vi "RT Main R1.vi"() -> ()   [LabVIEW 2018]
uses:
  Type Defs/Control Mode Type Def.ctl
  Type Defs/Sine Wave Inputs.ctl
  Type Defs/PID Inputs.ctl
  Type Defs/Measurement States.ctl
  <vilib>/Platform/TimedLoop/XDataNode/timing_clust.ctl
  <vilib>/Platform/TimedLoop/XDataNode/nitl_modes.ctl
  <vilib>/Platform/TimedLoop/XDataNode/wakeup.ctl
  <vilib>/FPGAPlugInAG/myRIO-1900/niLvFpga_Open_myRIO-1900.vi
  <vilib>/rvi/interface/common/dynamic/niFpgaDynamicAddResources.vi
  <vilib>/addons/control/pid/pid.llb/PID (DBL).vi
  <vilib>/Utility/error.llb/Error Cluster From Error Code.vi
  <vilib>/rvi/errors/niLvFpgaAdjustHostInterfaceError.vi
  <vilib>/FPGAPlugInAG/Dynamic/niLvFpga_Close_Dynamic.vi
  <vilib>/platform/TimedLoop/XDataNode/XDataNode.xnode
  <vilib>/rvi/interface/nirviOpenFPGA/nirviOpenFPGA.xnode
  FPGA Bitfiles/WattBalanceRev1_FPGATarget_FPGAMain_doRdIs9Lwbc.lvbitx
  FPGA/FPGA Main.vi
  <vilib>/rvi/interface/nirviReadWriteControl/nirviReadWriteControl.xnode
  <vilib>/rvi/interface/nirviCloseFPGA/nirviCloseFPGA.xnode
  <vilib>/rvi/interface/Simulation/niFpgaSimulationCallBeginRW.vi
  NiFpgaLv.dll
  <vilib>/Platform/TimedLoop/XDataNode/XDNodeRunTimeDep.lvlib
  <vilib>/addons/control/pid/NI_PID_pid.lvlib
panel:
  in  "Measure":bool
  out "Finished Late":bool
  in  "Amplifier On/Off":bool
  out "Voice Coil Input Voltage":dbl[](array[numeric]) format="%#.2g"
  out "Displacement (µm)":dbl[](array[numeric]) format="%#.2g"
  out "Voice Coil Back EMF":dbl[](array[numeric]) format="%#.2g"
  in  "PID Inputs":T1
  in  "Sine Wave\nInputs":T2
  in  "Manual Voice \nCoil Voltage":dbl format="%.2f"
  in  "Abort":bool
  in  "Control Mode":T3=enum."Manual"
  out "Chart":dynamicdata(graph) caption="Waveform Chart - dark"
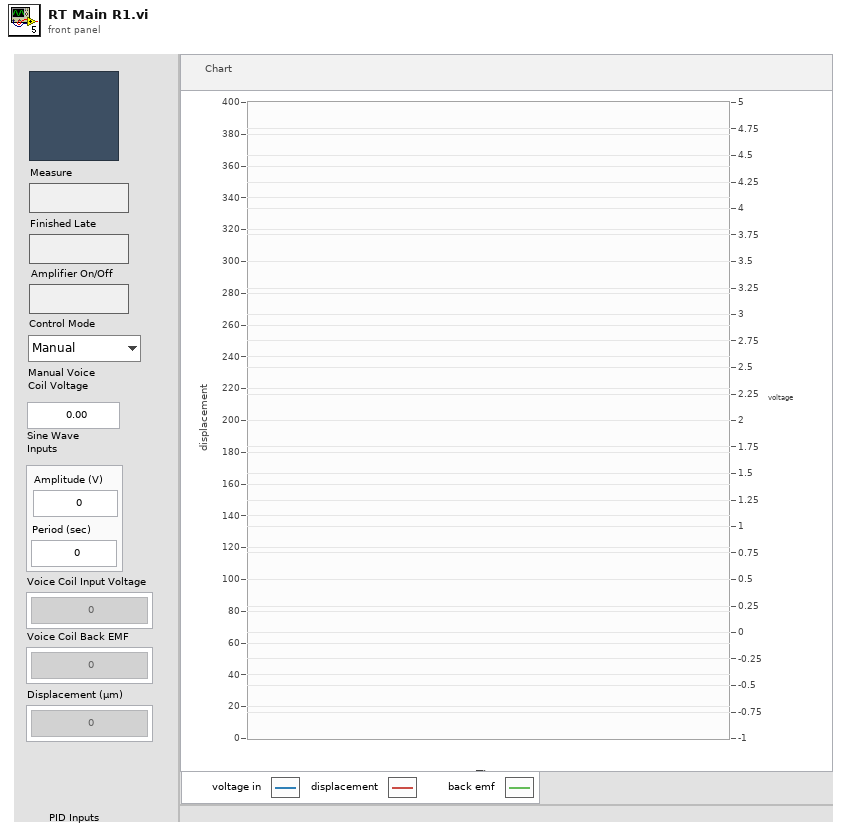
[diagram p1: front panel]
types:
  T1 = typedef "PID Inputs.ctl" = cluster{"PID":cluster{"Kp":dbl, "Ki":dbl, "Kd":dbl}, "Voltage Limits":cluster{"Max Voltage":dbl, "Min Voltage":dbl}, "Set Point (µm)":dbl}
  T2 = typedef "Sine Wave Inputs.ctl" = cluster{"Amplitude (V)":dbl, "Period (sec)":dbl}
  T3 = typedef "Control Mode Type Def.ctl" = enum16{"Sine", "PID", "Manual"}
  T4 = typedef "Measurement States.ctl" = enum16{"Idle", "Create File", "Collect Data", "Calculate", "Close"}
  T5 = typedef "XDNodeRunTimeDep.lvlib/timing_clust.ctl" = cluster{"Expected End [f-1]":u64, "Actual End [f-1]":u64, "Finished Late? [f-1]":bool, "Expected End [i-1]":u64, "Actual End [i-1]":u64, "Finished Late? [i-1]":bool, "Expected Start [i]":u64, "Actual Start [i]":u64, "Expected Start [f]":u64, "Actual Start [f]":u64, "Source Name":string, "Structure Name":string, "Period":i64, "Deadline":i64, "Offset":i64, "Start":i64, "Priority":i32, "Timeout":i32, "Mode":T6, "Wakeup Reason":T7, "Error":errorcluster, "Source Type":string, "Secondary Source Type":string, "Global End Time":u64, "Global Start Time":u64, "Frame Duration":u64, "Iteration Duration":u64, "Assigned CPU":i32, "I/O Scan Engine Mode":u32}
  T6 = typedef "XDNodeRunTimeDep.lvlib/nitl_modes.ctl" = enum32{"No Change", "Process missed periods, maintain original phase", "Discard missed periods, maintain original phase", "Process missed periods, ignore original phase", "Discard missed periods, ignore original phase"}
  T7 = typedef "XDNodeRunTimeDep.lvlib/wakeup.ctl" = enum32{"Normal", "Aborted", "Asynchronous wakeup", "Timing source error", "Timed loop error", "Timeout"}
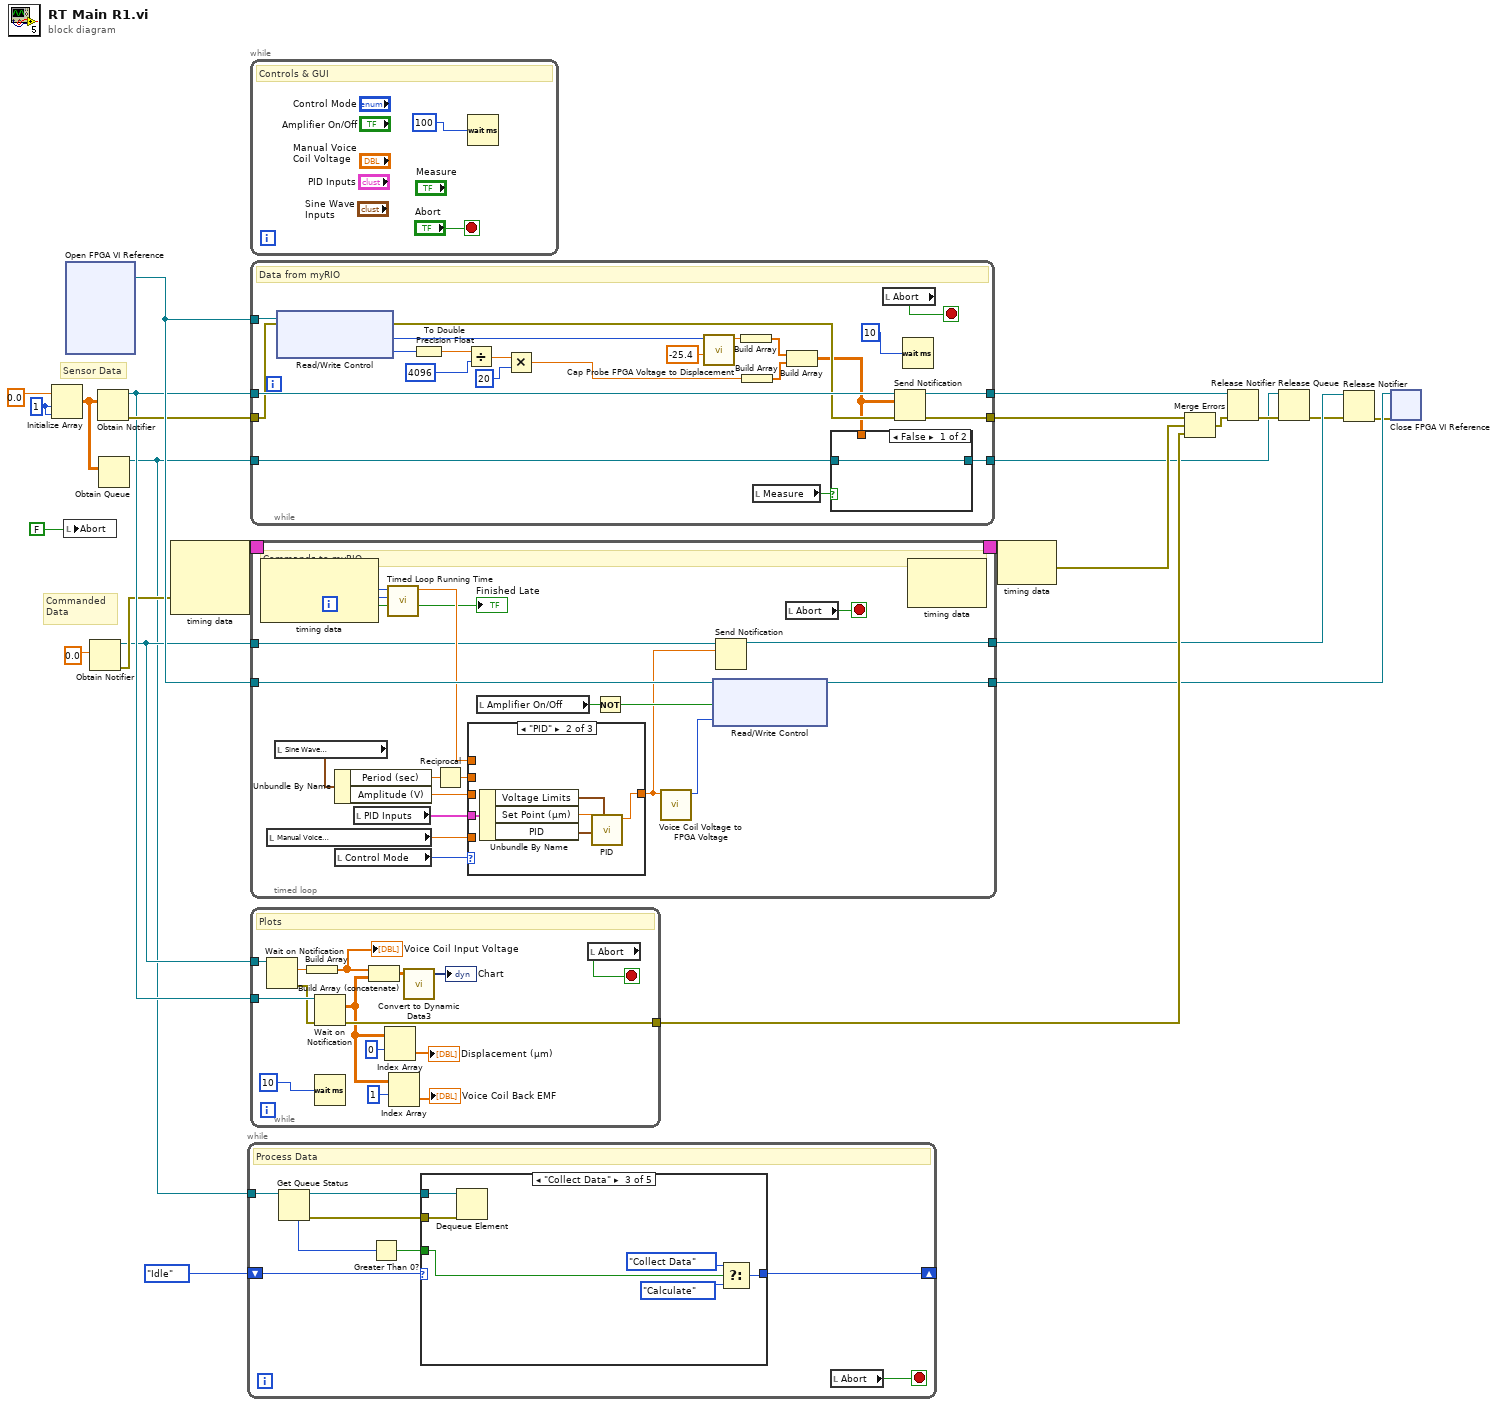
[diagram p0: block diagram]
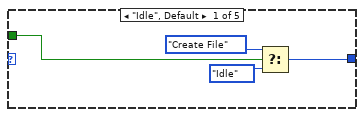
[diagram p2: hidden frame]
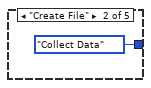
[diagram p3: hidden frame]
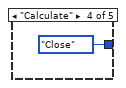
[diagram p4: hidden frame]
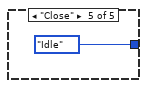
[diagram p5: hidden frame]
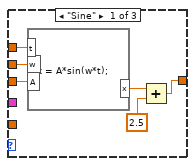
[diagram p6: hidden frame]
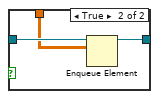
[diagram p8: hidden frame]
diagram:
  w21 = 1 ("dimension size")
  # "Commanded\nData"
  # "Sensor Data"
  n1 = Initialize Array(0.0, w21, w21) -> (w6:dbl[][])
  n2 = local write "Abort"(FALSE) -> ()
  n3 = xnode "Open FPGA VI Reference"() -> ("FPGA VI Reference Out"=w23:refnum<k20>)  [unwired: 2 in, 1 out]
  n4 = Obtain Notifier(notification data type=0.0) -> (notifier out=w11:refnum<notifier>, error out=w12:errorcluster)  [unwired: 3 in, 1 out]
  n5 = Obtain Notifier(notification data type=w6) -> (notifier out=w19:refnum<notifier>, error out=w20:errorcluster)  [unwired: 3 in, 1 out]
  n6 = Obtain Queue(element data type=w6) -> (queue out=w5:refnum<queue>)  [unwired: 4 in, 2 out]
  n7 = node-c288(w12) -> (w25:T5)  [unwired: 2 in]
  n8 = while {
    shift-right: [w28] -> _
    shift-left: Measurement_States."Idle" -> [w32]
    tunnel: w5 -> [w30]
    stop <- w33 stop-if-true
    # "Process Data"
    n9 = Get Queue Status(queue=w30) -> (queue out=w27:refnum<queue>, error out=w26:errorcluster, # elements in queue=w31:i32)  [unwired: 2 in, 5 out]
    n10 = Greater Than 0?(x=w31) -> (x > 0?=w29:bool)
    n11 = case shown="\"Collect Data\"" w32 {
      tunnel: w29 -> [w37 _ w44 _ _]
      tunnel: [w34 Measurement_States."Collect Data" w41 Measurement_States."Close" Measurement_States."Idle"] -> w28
      tunnel: w27 -> [_ _ w40 _ _]
      tunnel: w26 -> [_ _ w39 _ _]
      frame "Idle", Default {
        n12 = Select(t=Measurement_States."Create File", s=w37, f=Measurement_States."Idle") -> (s? t:f=w34:T4)
      }
      frame "Create File" {
      }
      frame "Collect Data" {
        n13 = Dequeue Element(queue=w40, error in (no error)=w39) -> ()  [unwired: 1 in, 4 out]
        n14 = Select(t=Measurement_States."Collect Data", s=w44, f=Measurement_States."Calculate") -> (s? t:f=w41:T4)
      }
      frame "Calculate" {
      }
      frame "Close" {
      }
    }
    n15 = local read "Abort"() -> (w33:bool)
  }
  n16 = while {
    stop <- "Abort" stop-if-true
    # "Controls & GUI"
    n17 = Wait (ms)(milliseconds to wait=100) -> ()  [unwired: 1 out]
  }
  n18 = while {
    tunnel: w23 -> [w70]
    tunnel: w19 -> [w63]
    tunnel: w20 -> [w62]
    tunnel: [w60] -> w14
    tunnel: [w59] -> w18
    tunnel: w5 -> [w51]
    tunnel: [w49] -> w2
    stop <- w67 stop-if-true
    # "Data from myRIO"
    n19 = xnode "Read/Write Control"("FPGA VI Reference In"=w70, "error in"=w62) -> ("error out"=w61:errorcluster, "Cap Probe Voltage"=w69:u16, "Read Coil"=w68:i16)  [unwired: 1 out]
    n20 = To Double Precision Float(number=w68) -> (double precision float=w57:dbl)
    n21 = Divide(x=w57, y=4096) -> (x/y=w55:dbl)
    n22 = Multiply(x=w55, y=20) -> (x*y=w53:dbl)
    n23 = call "Cap Probe FPGA Voltage to Displacement.vi"("Micrometers per Volt"=-25.4, "Cap Probe FPGA Voltage"=w69) -> ("Cap Probe Displacement"=w66:dbl)  [unwired: 9 in]
    n24 = Build Array(w66) -> (w65:dbl[])
    n25 = Build Array(w53) -> (w64:dbl[])
    n26 = local read "Measure"() -> (w52:bool)
    n27 = Build Array(w65, w64) -> (w50:dbl[][])
    n28 = case shown="False" w52 {
      tunnel: w51 -> [w72 w75]
      tunnel: w50 -> [_ w74]
      tunnel: [w72 w73] -> w49
      frame False {
      }
      frame True {
        n29 = Enqueue Element(queue=w75, element=w74) -> (queue out=w73:refnum<queue>)  [unwired: 2 in, 2 out]
      }
    }
    n30 = local read "Abort"() -> (w67:bool)
    n31 = Send Notification(notification=w50, notifier=w63, error in (no error)=w61) -> (notifier out=w60:refnum<notifier>, error out=w59:errorcluster)
    n32 = Wait (ms)(milliseconds to wait=10) -> ()  [unwired: 1 out]
  }
  n33 = timed-loop {
    timing: w25 -> [_]
    timing-out: [_] -> w24
    tunnel: w23 -> [w91]
    tunnel: [w86] -> w13
    tunnel: w11 -> [w79]
    tunnel: [w77] -> w9
    i -> [w83]
    stop <- w90 stop-if-true
    # "Commands to myRIO"
    n34 = node-c288() -> (w84:i64, →"Finished Late":bool)  [unwired: 1 in, 1 out]
    n35 = local read "Manual Voice \nCoil Voltage"() -> (w92:dbl)
    n36 = local read "Sine Wave\nInputs"() -> (w87:T2)
    n37 = Unbundle By Name(w87) -> ("Period (sec)"=w89:dbl, "Amplitude (V)"=w88:dbl)
    n38 = local read "Control Mode"() -> (w95:T3)
    n39 = local read "PID Inputs"() -> (w85:T1)
    n40 = call "Timed Loop Running Time.vi"("Counter"=w83, "Period (microsec)"=w84) -> ("Time (sec)"=w82:dbl)  [unwired: 9 in]
    n41 = Reciprocal(x=w89) -> (1/x=w93:dbl)
    n42 = case shown="\"PID\"" w95 {
      tunnel: w93 -> [w105 _ _]
      tunnel: w82 -> [w104 _ _]
      tunnel: [w102 w110 w111] -> w78
      tunnel: w92 -> [_ _ w111]
      tunnel: w88 -> [w100 _ _]
      tunnel: w85 -> [_ w109 _]
      frame "Sine" {
        n43 = formula code="x = A*sin(w*t);"("w"=w105, "t"=w104, "A"=w100) -> ("x"=w103:dbl)
        n44 = Add(x=w103, y=2.5) -> (x+y=w102:dbl)
      }
      frame "PID" {
        n45 = Unbundle By Name(w109) -> ("Voltage Limits"=w108:cluster{"Max Voltage":dbl, "Min Voltage":dbl}, "Set Point (µm)"=w107:dbl, "PID"=w106:cluster{"Kp":dbl, "Ki":dbl, "Kd":dbl})
        n46 = call-poly <vilib>:"PID.vi"("output range"=w108, "PID gains"=w106, "setpoint"=w107) -> ("output"=w110:dbl)  [unwired: 7 in, 1 out]
      }
      frame "Manual" {
      }
    }
    n47 = local read "Amplifier On/Off"() -> (w94:bool)
    n48 = Not(x=w94) -> (.not. x?=w81:bool)
    n49 = call "Voice Coil Voltage to FPGA Voltage.vi"("Voltage In"=w78) -> ("Voltage Out"=w80:u16)  [unwired: 10 in]
    n50 = xnode "Read/Write Control"("FPGA VI Reference In"=w91, "Amplifier On/Off"=w81, "Voice Coil Voltage"=w80) -> ("FPGA VI Reference Out"=w86:refnum<k20>)  [unwired: 1 in, 1 out]
    n51 = Send Notification(notification=w78, notifier=w79) -> (notifier out=w77:refnum<notifier>)  [unwired: 1 in, 1 out]
    n52 = local read "Abort"() -> (w90:bool)
    n53 = node-c288() -> ()  [unwired: 2 in, 1 out]
  }
  n54 = while {
    tunnel: w19 -> [w125]
    tunnel: [w119] -> w16
    tunnel: w11 -> [w118]
    stop <- w126 stop-if-true
    # "Plots"
    n55 = Wait on Notification(notifier=w118) -> (notification=w116:dbl, error out=w117:errorcluster)  [unwired: 3 in, 2 out]
    n56 = Build Array(w116) -> (w115:dbl[])
    "Voice Coil Input Voltage" <- w115
    n57 = Wait on Notification(notifier=w125, error in (no error)=w117) -> (notification=w113:dbl[][], error out=w119:errorcluster)  [unwired: 2 in, 2 out]
    n58 = Wait (ms)(milliseconds to wait=10) -> ()  [unwired: 1 out]
    n59 = Build Array (concatenate)(w115, w113) -> (w114:dbl[][])
    n60 = Index Array(array=w113, index (row)=0) -> (element=→"Displacement (µm)":dbl[])  [unwired: 1 in]
    n61 = Index Array(array=w113, index (row)=1) -> (element=→"Voice Coil Back EMF":dbl[])  [unwired: 1 in]
    n62 = call "Convert to Dynamic Data3"("2D Array"=w114) -> ("Dynamic Data Type"=→"Chart":dynamicdata)  [unwired: 3 in]
    n63 = local read "Abort"() -> (w126:bool)
  }
  n64 = node-c288(w24) -> (w17:errorcluster)
  n65 = Merge Errors(w18, w17, w16) -> (w15:errorcluster)
  n66 = Release Notifier(notifier=w14, error in (no error)=w15) -> (error out=w4:errorcluster)  [unwired: 1 in, 2 out]
  n67 = Release Queue(queue=w2, error in (no error)=w4) -> (error out=w3:errorcluster)  [unwired: 1 in, 2 out]
  n68 = Release Notifier(notifier=w9, error in (no error)=w3) -> (error out=w8:errorcluster)  [unwired: 1 in, 2 out]
  n69 = xnode "Close FPGA VI Reference"("FPGA VI Reference In"=w13, "error in"=w8) -> ()  [unwired: 1 out]
